vi "RSW_cluster.vi"() -> ()   [LabVIEW 2015]
doc: "Reading an ini file, sorting using a cluster, writing sorted data to a new ini file."
uses:
  <vilib>/Utility/config.llb/Read Key (String).vi
  <vilib>/Utility/config.llb/Write Key (String).vi
  <vilib>/Utility/config.llb/NI_LVConfig.lvlib
panel:
  out "sorted array":T1(array[cluster])
  out "error out":errorcluster
  in  "Sorted ini file":path
  in  "The path of the ini file":path
  in  "Cluster":T2
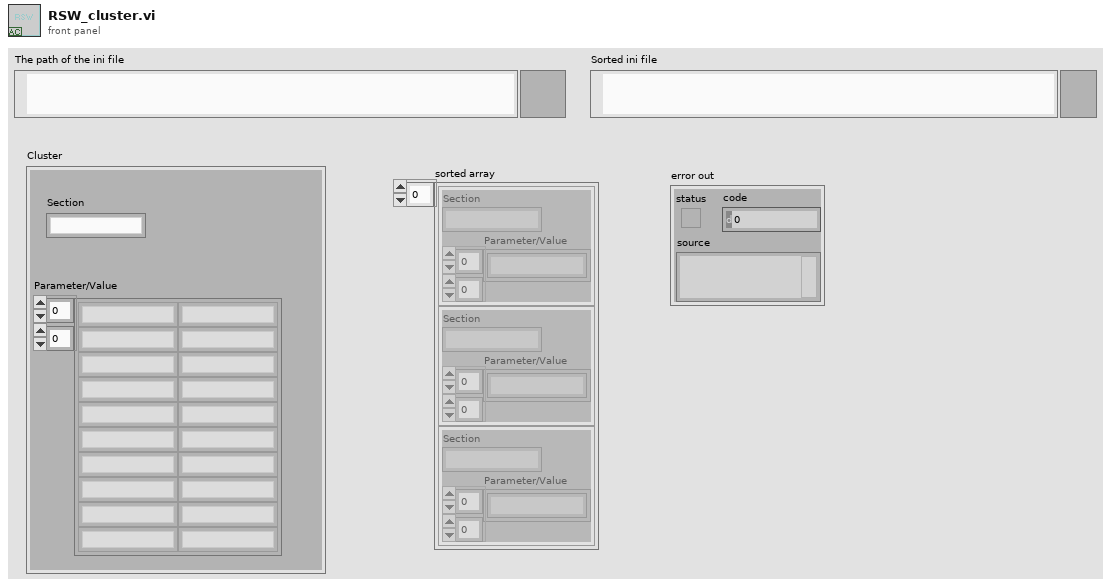
[diagram p1: front panel]
types:
  T1 = cluster{"Section":string, "Parameter/Value":string[][]}[]
  T2 = cluster{"Section":string, "Parameter/Value":string[][]}
  T3 = typedef "NI_LVConfig.lvlib/Config Data RefNum.ctl" = refnum<k1>
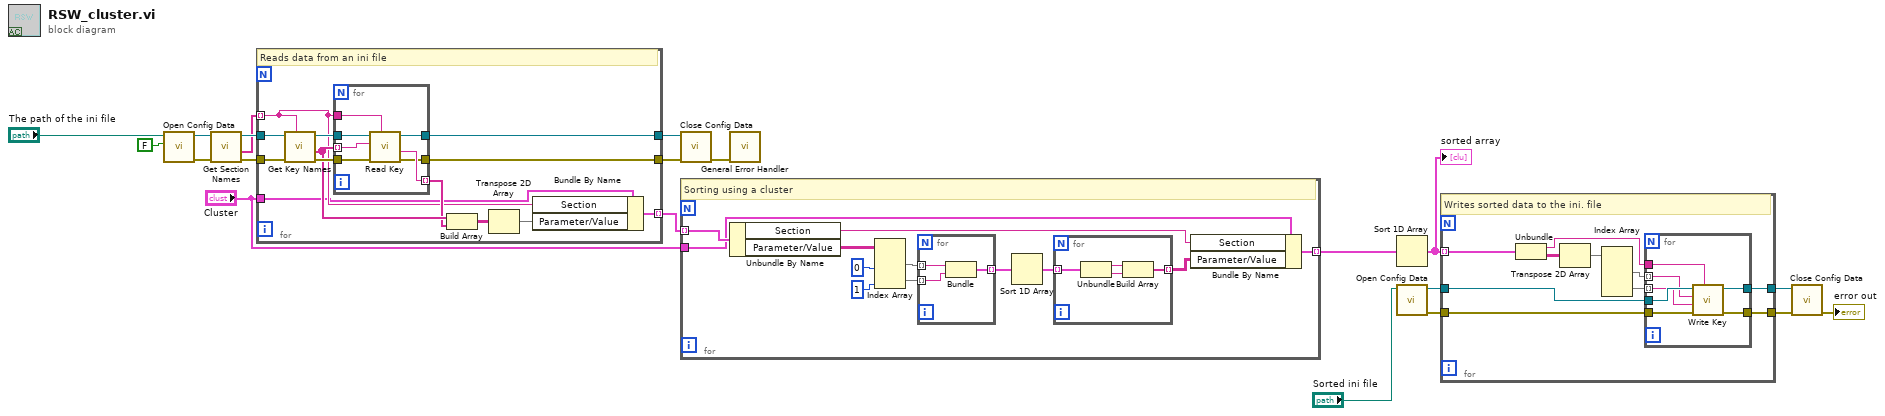
[diagram p0: block diagram]
diagram:
  n1 = call <vilib>:"Open Config Data.vi"("create file if necessary (T)"=FALSE, "configuration file path"="The path of the ini file") -> ("error out"=w19:errorcluster, "refnum"=w20:T3)  [unwired: 7 in, 1 out]
  n2 = call <vilib>:"Get Section Names.vi"("error in (no error)"=w19, "refnum"=w20) -> ("error out"=w17:errorcluster, "section names"=w16:string[], "refnum out"=w18:T3)  [unwired: 7 in]
  n3 = for {
    tunnel: w16 -> [w26] mode=indexing
    tunnel: w18 -> [w32]
    tunnel: w17 -> [w33]
    tunnel: [w25] -> w2 mode=indexing
    tunnel: "Cluster" -> [w24]
    tunnel: [w22] -> w11
    tunnel: [w21] -> w10
    # "Reads data from an ini file"
    n4 = call <vilib>:"Get Key Names.vi"("section"=w26, "error in (no error)"=w33, "refnum"=w32) -> ("error out"=w31:errorcluster, "key names"=w29:string[], "refnum out"=w30:T3)  [unwired: 5 in, 1 out]
    n5 = for {
      tunnel: w26 -> [w40]
      tunnel: w29 -> [w39] mode=indexing
      tunnel: w30 -> [w38]
      tunnel: w31 -> [w37]
      tunnel: [w36] -> w28 mode=indexing
      tunnel: [w35] -> w21
      tunnel: [w34] -> w22
      n6 = call-poly <vilib>:"Read Key.vi"("section"=w40, "error in (no error)"=w37, "key"=w39, "refnum"=w38) -> ("error out"=w34:errorcluster, "value"=w36:string, "refnum out"=w35:T3)  [unwired: 4 in, 1 out]
    }
    n7 = Build Array(w29, w28) -> (w27:string[][])
    n8 = Transpose 2D Array(2D array=w27) -> (transposed array=w23:string[][])
    n9 = Bundle By Name(cluster=w24, "Section"=w26, "Parameter/Value"=w23) -> (w25:T2)
  }
  n10 = call <vilib>:"Close Config Data.vi"("error in (no error)"=w11, "refnum"=w10) -> ("error out"=w12:errorcluster)  [unwired: 8 in, 1 out]
  n11 = for {
    tunnel: w2 -> [w52] mode=indexing
    tunnel: "Cluster" -> [w51]
    tunnel: [w50] -> w1 mode=indexing
    # "Sorting using a cluster"
    n12 = Unbundle By Name(w52) -> ("Section"=w49:string, "Parameter/Value"=w42:string[][])
    n13 = Index Array(array=w42, index (col) #1=0, index (col) #2=1) -> (element #1=w46:string[], element #2=w45:string[])  [unwired: 2 in]
    n14 = for {
      tunnel: w46 -> [w59] mode=indexing
      tunnel: w45 -> [w58] mode=indexing
      tunnel: [w57] -> w44 mode=indexing
      n15 = Bundle("String"=w59, "String"=w58) -> (w57:cluster{"String":string, "String":string})  [unwired: 1 in]
    }
    n16 = Sort 1D Array(array=w44) -> (sorted array=w43:cluster{"String":string, "String":string}[])
    n17 = for {
      tunnel: w43 -> [w56] mode=indexing
      tunnel: [w53] -> w41 mode=indexing
      n18 = Unbundle(w56) -> ("String"=w55:string, "String"=w54:string)
      n19 = Build Array(w55, w54) -> (w53:string[])
    }
    n20 = Bundle By Name(cluster=w51, "Section"=w49, "Parameter/Value"=w41) -> (w50:T2)
  }
  n21 = call <vilib>:"General Error Handler.vi"("error in (no error)"=w12) -> ()  [unwired: 10 in, 5 out]
  n22 = Sort 1D Array(array=w1) -> (sorted array=w9:T1)
  "sorted array" <- w9
  n23 = call <vilib>:"Open Config Data.vi"("configuration file path"="Sorted ini file") -> ("error out"=w7:errorcluster, "refnum"=w8:T3)  [unwired: 8 in, 1 out]
  n24 = for {
    tunnel: w9 -> [w69] mode=indexing
    tunnel: w8 -> [w67]
    tunnel: w7 -> [w65]
    tunnel: [w64] -> w6
    tunnel: [w63] -> w5
    # "Writes sorted data to the ini. file"
    n25 = Unbundle(w69) -> ("Section"=w68:string, "Parameter/Value"=w62:string[][])
    n26 = Transpose 2D Array(2D array=w62) -> (transposed array=w61:string[][])
    n27 = Index Array(array=w61) -> (element #1=w66:string[], element #2=w60:string[])  [unwired: 4 in]
    n28 = for {
      tunnel: w68 -> [w76]
      tunnel: w67 -> [w75]
      tunnel: w66 -> [w73] mode=indexing
      tunnel: w65 -> [w74]
      tunnel: [w71] -> w64
      tunnel: [w72] -> w63
      tunnel: w60 -> [w70] mode=indexing
      n29 = call-poly <vilib>:"Write Key.vi"("section"=w76, "error in (no error)"=w74, "value"=w70, "key"=w73, "refnum"=w75) -> ("error out"=w71:errorcluster, "refnum out"=w72:T3)  [unwired: 4 in, 1 out]
    }
  }
  n30 = call <vilib>:"Close Config Data.vi"("error in (no error)"=w6, "refnum"=w5) -> ("error out"=→"error out":errorcluster)  [unwired: 8 in, 1 out]
